vi "Preset subsystems.vi"(9 "Claw Angle":dbl, 10 "Arm Extend?":bool, 11 "Arm Angle":dbl) -> ()   [LabVIEW 2017]
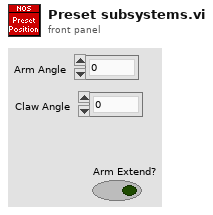
[diagram p1: front panel]
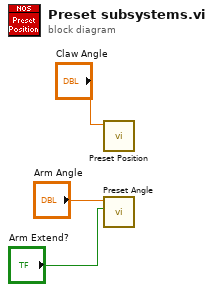
[diagram p0: block diagram]
diagram:
  n1 = call "Preset Position.vi"("Preset Angle"="Claw Angle") -> ()  [unwired: 10 in, 1 out]
  n2 = call "Preset Angle.vi"("Arm Out?"="Arm Extend?", "Setpoint"="Arm Angle") -> ()  [unwired: 9 in, 1 out]
